vi "set method 2.vi"(1 "seconds/data point":u16=10 min=1 max=9999 step=1, 2 "ok":bool, 3 "auto/manual":bool, 4 "Channel A":enum16{"OFF", "pH", "mV", "ion", "conductivity"}(ring)=enum."pH", 5 "Channel B":enum16{"OFF", "pH", "mV", "ion"}(ring)) -> (14 "canceled":bool=TRUE, 15 "seconds/data point out":u16=10 min=1 max=9999 step=1, 16 "2nd channel":bool=TRUE, 17 "auto/manual out":bool=TRUE, 18 "Channel A out":enum16{"OFF", "pH", "mV", "ion", "conductivity"}(ring)=enum."pH", 19 "Channel B out":enum16{"OFF", "pH", "mV", "ion"}(ring)=enum."pH")   [LabVIEW 2010]
panel:
  out "setting up meter":string="Sending method to meter. Please wait. Do not change the display of the meter after setting the method!"
  in  "probe type":string[](array[string])=["", "A", "B", "C", "D"]
  in  "cancel":bool
  out "channels":T1(ring)
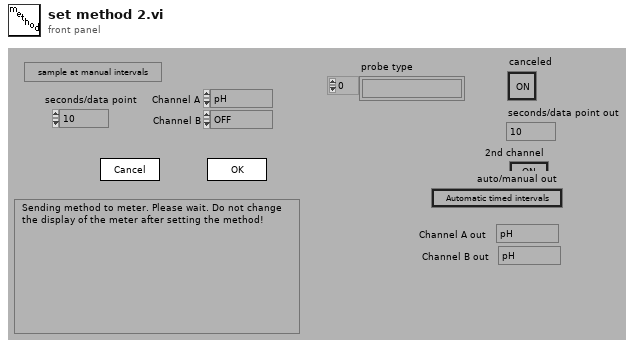
[diagram p1: front panel]
types:
  T1 = enum16{"channel A", "Channel B", "Channel A and B"}
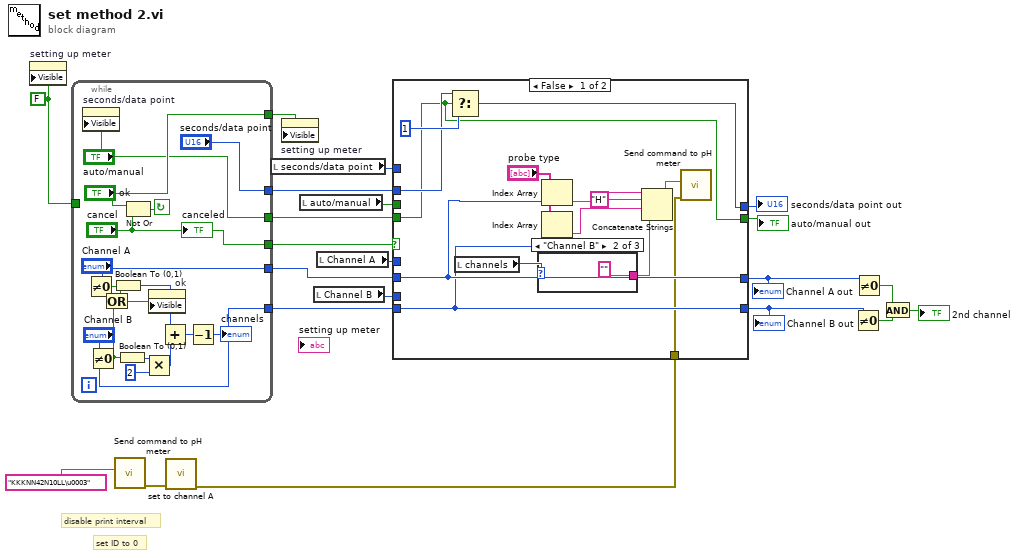
[diagram p0: block diagram]
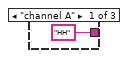
[diagram p2: hidden frame]
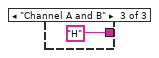
[diagram p3: hidden frame]
diagram:
  w5 = FALSE
  # "set ID to 0"
  # "disable print interval"
  n1 = property on="setting up meter" class="Str"("Visible"=w5) -> ()  [unwired: 2 in, 2 out]
  n2 = while {
    tunnel: ["ok"] -> w3
    tunnel: w5 -> [_]
    tunnel: ["Channel B"] -> w11
    tunnel: ["Channel A"] -> w12
    tunnel: ["auto/manual"] -> w15
    tunnel: ["seconds/data point"] -> w19
    tunnel: ["cancel"] -> w21
    stop <- w22 continue-if-true
    n3 = property on="seconds/data point" class="DigNum (strict)"("Visible"="auto/manual") -> ()  [unwired: 2 in, 2 out]
    n4 = Not Equal To 0?(x="Channel A") -> (x != 0?=w25:bool)
    n5 = Not Equal To 0?(x="Channel B") -> (x != 0?=w24:bool)
    n6 = Or(x=w25, y=w24) -> (x .or. y?=w26:bool)
    n7 = Boolean To (0,1)(Boolean=w25) -> (0, 1=w27:i16)
    n8 = Boolean To (0,1)(Boolean=w24) -> (0, 1=w30:i16)
    n9 = Not Or(1:"cancel", 2:"ok") -> (0:w22:bool)
    n10 = Multiply(x=w30, y=2) -> (x*y=w29:i32)
    n11 = property on="ok" class="Bool"("Visible"=w26) -> ()  [unwired: 2 in, 2 out]
    n12 = Add(x=w27, y=w29) -> (x+y=w34:i32)
    n13 = Decrement(x=w34) -> (x-1=→"channels":i32)
    "canceled" <- "cancel"
  }
  n14 = call "Send command to pH meter"("string to write"="KKKNN42N10LL\u0003") -> ("error out"=w2:errorcluster)  [unwired: 9 in, 1 out]
  n15 = call "set to channel A.vi"("error in (no error)"=w2) -> ("error out"=w1:errorcluster)  [unwired: 10 in]
  n16 = local read "seconds/data point"() -> (w16:u16)
  n17 = property on="setting up meter" class="Str"("Visible"=w3) -> ()  [unwired: 2 in, 2 out]
  n18 = local read "auto/manual"() -> (w13:bool)
  n19 = local read "Channel B"() -> (w9:enum16{"OFF", "pH", "mV", "ion"})
  n20 = local read "Channel A"() -> (w10:enum16{"OFF", "pH", "mV", "ion", "conductivity"})
  n21 = case shown="False" w21 {
    tunnel: [w39 w58] -> w20
    tunnel: w19 -> [w41 _]
    tunnel: w16 -> [_ w58]
    tunnel: w15 -> [w40 _]
    tunnel: [w40 w57] -> w14
    tunnel: w13 -> [_ w57]
    tunnel: w12 -> [w51 _]
    tunnel: w11 -> [w50 _]
    tunnel: [w51 w56] -> w6
    tunnel: w10 -> [_ w56]
    tunnel: [w50 w55] -> w7
    tunnel: w9 -> [_ w55]
    tunnel: w1 -> [w38 _]
    frame False {
      n22 = Select(t=w41, s=w40, f=u16 1) -> (s? t:f=w39:u16)
      n23 = local read "channels"() -> (w47:T1)
      n24 = case shown="\"Channel B\"" w47 {
        tunnel: ["HH" "" "H"] -> w46
        frame "channel A" {
        }
        frame "Channel B" {
        }
        frame "Channel A and B" {
        }
      }
      n25 = Index Array(array="probe type", index=w51) -> (element=w42:string)
      n26 = Index Array(array="probe type", index=w50) -> (element=w44:string)
      n27 = Concatenate Strings(w42, "H", w44, w46) -> (w48:string)
      n28 = call "Send command to pH meter"("error in (no error)"=w38, "string to write"=w48) -> ()  [unwired: 8 in, 2 out]
    }
    frame True {
    }
  }
  "seconds/data point out" <- w20
  "Channel A out" <- w6
  "Channel B out" <- w7
  "auto/manual out" <- w14
  n29 = Not Equal To 0?(x=w7) -> (x != 0?=w18:bool)
  n30 = Not Equal To 0?(x=w6) -> (x != 0?=w17:bool)
  n31 = And(x=w17, y=w18) -> (x .and. y?=→"2nd channel":bool)
